vi "Utils - Convert1DImageToImaqImage.vi"(6 "Image In":T3, 8 "error in (no error)":errorcluster, 9 "1DImageData In":u8[](array[numeric]), 11 "Image Properties In":T1) -> (0 "error out":errorcluster, 1 "1DImageData Out":u8[](array[numeric]), 4 "Image Out":T3)   [LabVIEW 2015]
doc: "Convert 1d U8 Image array to LabVIEW image. This VI supports only Mono8 image format."
uses:
  <vilib>/vision/NI_Vision_Development_Module.lvlib
  PRM/IMG_FORMAT/IMG_DATA_FORMAT.ctl
  xiImageManager/xiImageMng - Attributes.ctl
  <vilib>/vision/Image Controls.llb/IMAQ Image.ctl
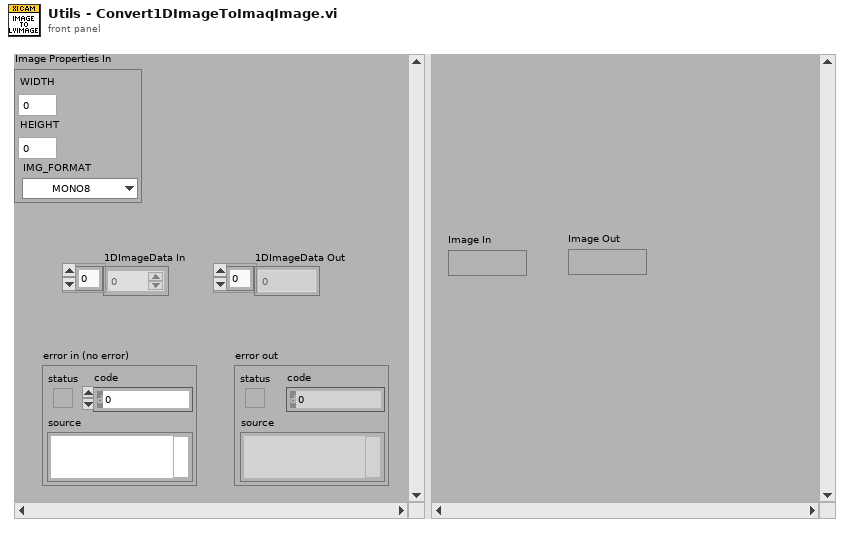
[diagram p1: front panel]
types:
  T1 = typedef "xiImageMng - Attributes.ctl" = cluster{"WIDTH":i32, "HEIGHT":i32, "IMG_FORMAT":T2}
  T2 = typedef "IMG_DATA_FORMAT.ctl" = enum16{"MONO8", "MONO16", "RGB24", "RGB32", "RGBPLANAR", "RAW8", "RAW16"}
  T3 = typedef "IMAQ Image.ctl" = refnum<image>
  T4 = typedef "Image Type" = u32
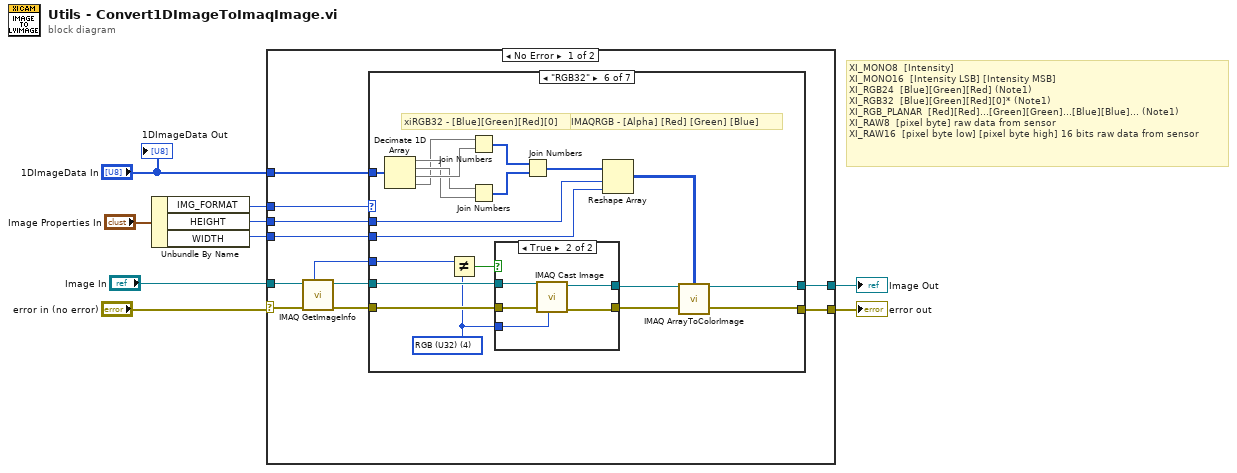
[diagram p0: block diagram]
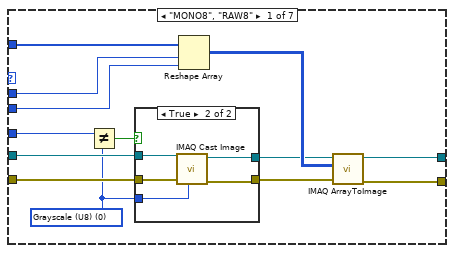
[diagram p2: hidden frame]
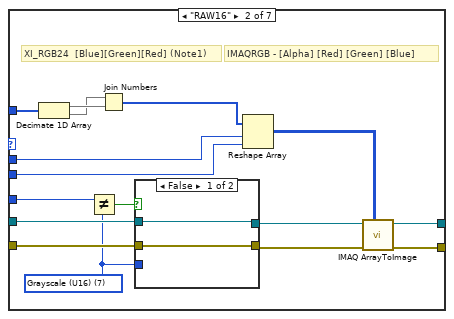
[diagram p4: hidden frame]
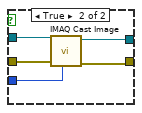
[diagram p5: hidden frame]
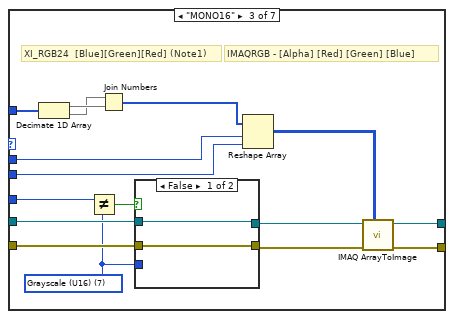
[diagram p6: hidden frame]
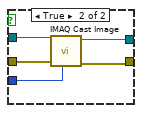
[diagram p7: hidden frame]
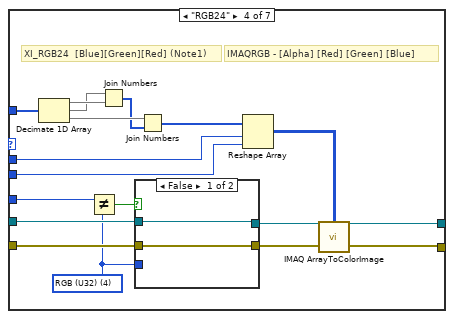
[diagram p8: hidden frame]
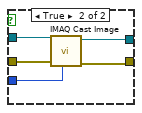
[diagram p9: hidden frame]
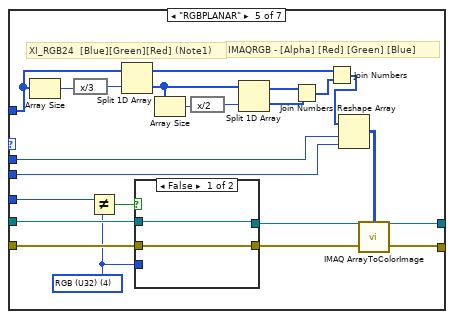
[diagram p10: hidden frame]
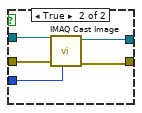
[diagram p11: hidden frame]
diagram:
  # "XI_MONO8\t [Intensity]\nXI_MONO16\t [Intensity LSB] [Intensity MSB]\nXI_RGB24\t [Blue][Green][Red] (Note1)\nXI_RGB32\t [Blue][Green][Red][0]* (Note1)\nXI_RGB_PLANAR\t [Red][Red]...[Green][Green]...[Blue][Blue]... (Note1)\nXI_RAW8\t [pixel byte] raw data from sensor\t\nXI_RAW16\t [pixel byte low] [pixel byte high] 16 bits raw data from sensor"
  n1 = Unbundle By Name("Image Properties In") -> ("IMG_FORMAT"=w6:T2, "HEIGHT"=w5:i32, "WIDTH"=w4:i32)
  n2 = case shown="No Error" "error in (no error)" {
    selector: "error in (no error)" -> [w16 w170]
    tunnel: "1DImageData In" -> [w19 _]
    tunnel: w6 -> [w10 _]
    tunnel: w5 -> [w18 _]
    tunnel: w4 -> [w17 _]
    tunnel: "Image In" -> [w13 w171]
    tunnel: [w12 w171] -> w1
    tunnel: [w11 w170] -> w2
    frame No Error {
      n3 = call "IMAQ GetImageInfo"("error in (no error)"=w16, "Image"=w13) -> ("error out"=w15:errorcluster, "Image Type"=w14:T4)  [unwired: 2 in, 6 out]
      n4 = case shown="\"RGB32\"" w10 {
        tunnel: w19 -> [w32 w46 w69 w87 w119 w153 _]
        tunnel: w18 -> [w31 w55 w78 w103 w133 w160 _]
        tunnel: w17 -> [w30 w54 w77 w102 w132 w159 _]
        tunnel: w15 -> [w26 w50 w73 w98 w128 w155 w168]
        tunnel: w14 -> [w29 w53 w76 w101 w131 w158 _]
        tunnel: w13 -> [w27 w51 w74 w99 w129 w156 w169]
        tunnel: [w21 w44 w67 w93 w123 w149 w169] -> w12
        tunnel: [w20 w43 w66 w92 w122 w148 w168] -> w11
        frame "MONO8", "RAW8" {
          w25 = T4 0 items=["Grayscale (U8)", "Grayscale (I16)", "Grayscale (SGL)", "Complex (CSG)", "RGB (U32)", "HSL (U32)", "RGB (U64)", "Grayscale (U16)"] ("Image Type")
          n5 = Not Equal?(x=w29, y=w25) -> (x != y?=w28:bool)
          n6 = case shown="True" w28 {
            tunnel: w27 -> [w33 w39]
            tunnel: w26 -> [w34 w38]
            tunnel: w25 -> [_ w37]
            tunnel: [w33 w36] -> w23
            tunnel: [w34 w35] -> w22
            frame False {
            }
            frame True {
              n7 = call "IMAQ Cast Image"("Image Type"=w37, "error in (no error)"=w38, "Image Src"=w39) -> ("error out"=w35:errorcluster, "Image Dst Out"=w36:T3)  [unwired: 7 in]
            }
          }
          n8 = Reshape Array(w32, w31, w30) -> (w24:u8[][])
          n9 = call "IMAQ ArrayToImage"("error in (no error)"=w22, "Image Pixels (U8)"=w24, "Image"=w23) -> ("error out"=w20:errorcluster, "Image Out"=w21:T3)  [unwired: 7 in]
        }
        frame "RAW16" {
          w49 = T4 7 items=["Grayscale (U8)", "Grayscale (I16)", "Grayscale (SGL)", "Complex (CSG)", "RGB (U32)", "HSL (U32)", "RGB (U64)", "Grayscale (U16)"] ("Image Type")
          # "IMAQRGB - [Alpha] [Red] [Green] [Blue]"
          # "XI_RGB24\t [Blue][Green][Red] (Note1)"
          n10 = Decimate 1D Array(w46) -> (w48:u8[], w47:u8[])
          n11 = Not Equal?(x=w53, y=w49) -> (x != y?=w52:bool)
          n12 = Join Numbers(hi=w47, lo=w48) -> ((hi.lo)=w45:u16[])
          n13 = case shown="False" w52 {
            tunnel: w51 -> [w56 w62]
            tunnel: w50 -> [w57 w61]
            tunnel: w49 -> [_ w60]
            tunnel: [w56 w59] -> w41
            tunnel: [w57 w58] -> w42
            frame False {
            }
            frame True {
              n14 = call "IMAQ Cast Image"("Image Type"=w60, "error in (no error)"=w61, "Image Src"=w62) -> ("error out"=w58:errorcluster, "Image Dst Out"=w59:T3)  [unwired: 7 in]
            }
          }
          n15 = Reshape Array(w45, w55, w54) -> (w40:u16[][])
          n16 = call "IMAQ ArrayToImage"("Image Pixels (U16)"=w40, "error in (no error)"=w42, "Image"=w41) -> ("error out"=w43:errorcluster, "Image Out"=w44:T3)  [unwired: 7 in]
        }
        frame "MONO16" {
          w72 = T4 7 items=["Grayscale (U8)", "Grayscale (I16)", "Grayscale (SGL)", "Complex (CSG)", "RGB (U32)", "HSL (U32)", "RGB (U64)", "Grayscale (U16)"] ("Image Type")
          # "IMAQRGB - [Alpha] [Red] [Green] [Blue]"
          # "XI_RGB24\t [Blue][Green][Red] (Note1)"
          n17 = Decimate 1D Array(w69) -> (w71:u8[], w70:u8[])
          n18 = Not Equal?(x=w76, y=w72) -> (x != y?=w75:bool)
          n19 = Join Numbers(hi=w70, lo=w71) -> ((hi.lo)=w68:u16[])
          n20 = case shown="False" w75 {
            tunnel: w74 -> [w79 w85]
            tunnel: w73 -> [w80 w84]
            tunnel: w72 -> [_ w83]
            tunnel: [w79 w82] -> w64
            tunnel: [w80 w81] -> w65
            frame False {
            }
            frame True {
              n21 = call "IMAQ Cast Image"("Image Type"=w83, "error in (no error)"=w84, "Image Src"=w85) -> ("error out"=w81:errorcluster, "Image Dst Out"=w82:T3)  [unwired: 7 in]
            }
          }
          n22 = Reshape Array(w68, w78, w77) -> (w63:u16[][])
          n23 = call "IMAQ ArrayToImage"("Image Pixels (U16)"=w63, "error in (no error)"=w65, "Image"=w64) -> ("error out"=w66:errorcluster, "Image Out"=w67:T3)  [unwired: 7 in]
        }
        frame "RGB24" {
          w97 = T4 4 items=["Grayscale (U8)", "Grayscale (I16)", "Grayscale (SGL)", "Complex (CSG)", "RGB (U32)", "HSL (U32)", "RGB (U64)", "Grayscale (U16)"] ("Image Type")
          # "IMAQRGB - [Alpha] [Red] [Green] [Blue]"
          # "XI_RGB24\t [Blue][Green][Red] (Note1)"
          n24 = Decimate 1D Array(w87) -> (w90:u8[], w89:u8[], w91:u8[])
          n25 = Not Equal?(x=w101, y=w97) -> (x != y?=w100:bool)
          n26 = Join Numbers(hi=w89, lo=w90) -> ((hi.lo)=w88:u16[])
          n27 = case shown="False" w100 {
            tunnel: w99 -> [w104 w110]
            tunnel: w98 -> [w105 w109]
            tunnel: w97 -> [_ w108]
            tunnel: [w104 w107] -> w96
            tunnel: [w105 w106] -> w94
            frame False {
            }
            frame True {
              n28 = call "IMAQ Cast Image"("Image Type"=w108, "error in (no error)"=w109, "Image Src"=w110) -> ("error out"=w106:errorcluster, "Image Dst Out"=w107:T3)  [unwired: 7 in]
            }
          }
          n29 = Join Numbers(hi=w91, lo=w88) -> ((hi.lo)=w86:u32[])
          n30 = Reshape Array(w86, w103, w102) -> (w95:u32[][])
          n31 = call "IMAQ ArrayToColorImage"("Image Pixels (U32)"=w95, "Image"=w96, "error in (no error)"=w94) -> ("Image Out"=w93:T3, "error out"=w92:errorcluster)  [unwired: 2 in]
        }
        frame "RGBPLANAR" {
          w127 = T4 4 items=["Grayscale (U8)", "Grayscale (I16)", "Grayscale (SGL)", "Complex (CSG)", "RGB (U32)", "HSL (U32)", "RGB (U64)", "Grayscale (U16)"] ("Image Type")
          # "IMAQRGB - [Alpha] [Red] [Green] [Blue]"
          # "XI_RGB24\t [Blue][Green][Red] (Note1)"
          n32 = Array Size(array=w119) -> (size(s)=w120:i32)
          n33 = expression code="x/3"(w120) -> (w121:i32)
          n34 = Not Equal?(x=w131, y=w127) -> (x != y?=w130:bool)
          n35 = Split 1D Array(array=w119, index=w121) -> (first subarray=w118:u8[], second subarray=w115:u8[])
          n36 = case shown="False" w130 {
            tunnel: w129 -> [w134 w140]
            tunnel: w128 -> [w135 w139]
            tunnel: w127 -> [_ w138]
            tunnel: [w134 w137] -> w126
            tunnel: [w135 w136] -> w124
            frame False {
            }
            frame True {
              n37 = call "IMAQ Cast Image"("Image Type"=w138, "error in (no error)"=w139, "Image Src"=w140) -> ("error out"=w136:errorcluster, "Image Dst Out"=w137:T3)  [unwired: 7 in]
            }
          }
          n38 = Array Size(array=w115) -> (size(s)=w117:i32)
          n39 = expression code="x/2"(w117) -> (w116:i32)
          n40 = Split 1D Array(array=w115, index=w116) -> (first subarray=w114:u8[], second subarray=w113:u8[])
          n41 = Join Numbers(hi=w114, lo=w113) -> ((hi.lo)=w112:u16[])
          n42 = Join Numbers(hi=w118, lo=w112) -> ((hi.lo)=w111:u32[])
          n43 = Reshape Array(w111, w133, w132) -> (w125:u32[][])
          n44 = call "IMAQ ArrayToColorImage"("Image Pixels (U32)"=w125, "Image"=w126, "error in (no error)"=w124) -> ("Image Out"=w123:T3, "error out"=w122:errorcluster)  [unwired: 2 in]
        }
        frame "RGB32" {
          w154 = T4 4 items=["Grayscale (U8)", "Grayscale (I16)", "Grayscale (SGL)", "Complex (CSG)", "RGB (U32)", "HSL (U32)", "RGB (U64)", "Grayscale (U16)"] ("Image Type")
          # "IMAQRGB - [Alpha] [Red] [Green] [Blue]"
          # "xiRGB32 - [Blue][Green][Red][0]"
          n45 = Decimate 1D Array(w153) -> (w143:u8[], w144:u8[], w145:u8[], w141:u8[])
          n46 = Not Equal?(x=w158, y=w154) -> (x != y?=w157:bool)
          n47 = Join Numbers(hi=w141, lo=w145) -> ((hi.lo)=w147:u16[])
          n48 = Join Numbers(hi=w144, lo=w143) -> ((hi.lo)=w146:u16[])
          n49 = case shown="True" w157 {
            tunnel: w156 -> [w161 w167]
            tunnel: w155 -> [w162 w166]
            tunnel: w154 -> [_ w165]
            tunnel: [w161 w164] -> w152
            tunnel: [w162 w163] -> w150
            frame False {
            }
            frame True {
              n50 = call "IMAQ Cast Image"("Image Type"=w165, "error in (no error)"=w166, "Image Src"=w167) -> ("error out"=w163:errorcluster, "Image Dst Out"=w164:T3)  [unwired: 7 in]
            }
          }
          n51 = Join Numbers(hi=w147, lo=w146) -> ((hi.lo)=w142:u32[])
          n52 = Reshape Array(w142, w160, w159) -> (w151:u32[][])
          n53 = call "IMAQ ArrayToColorImage"("Image Pixels (U32)"=w151, "Image"=w152, "error in (no error)"=w150) -> ("Image Out"=w149:T3, "error out"=w148:errorcluster)  [unwired: 2 in]
        }
        frame Default {
        }
      }
    }
    frame Error {
    }
  }
  "error out" <- w2
  "Image Out" <- w1
  "1DImageData Out" <- "1DImageData In"
